vi "Add to Tree.vi"(8 "error in":errorcluster, 11 "Data in":T1) -> (0 "error out":errorcluster, 3 "Data out":T1)   [LabVIEW 2020, in "Peek Window.lvlib"]
uses:
  Peek Window.lvlib
  MHL Data Cluster.ctl
  Open Diagram Argument--cluster.ctl
  VI Types Enum.ctl
  Symbols Enum.ctl
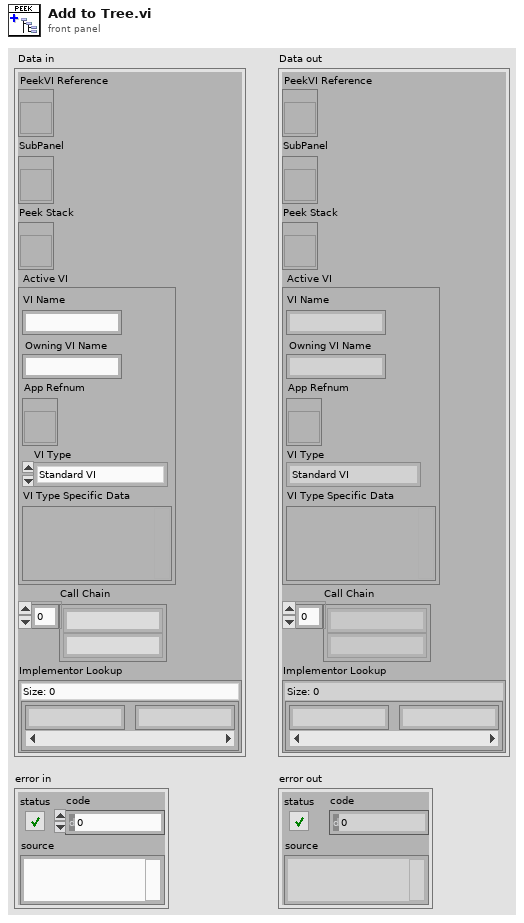
[diagram p1: front panel]
types:
  T1 = typedef "Peek Window.lvlib/MHL Data Cluster.ctl" = cluster{"PeekVI Reference":refnum<vi>, "SubPanel":refnum<vi>, "Peek Stack":refnum<vi>, "Active VI":T2, "Call Chain":string[], "Implementor Lookup":map{string, string}}
  T2 = typedef "Peek Window.lvlib/Open Diagram Argument--cluster.ctl" = cluster{"VI Name":string, "Owning VI Name":string, "App Refnum":refnum<vi>, "VI Type":T3, "VI Type Specific Data":variant}
  T3 = typedef "Peek Window.lvlib/VI Types Enum.ctl" = enum16{"Standard VI", "Dynamic Dispatch VI", "Malleable VI", "Express VI", "Polymorphic VI", "Missing VI"}
  T4 = typedef "Peek Window.lvlib/Symbols Enum.ctl" = enum16{"<Blank>", "Below Here Glyph", "VI", "Dynamic Dispatch VI", "Malleable VI", "Polymorphic VI", "Missing VI", "Express VI"}
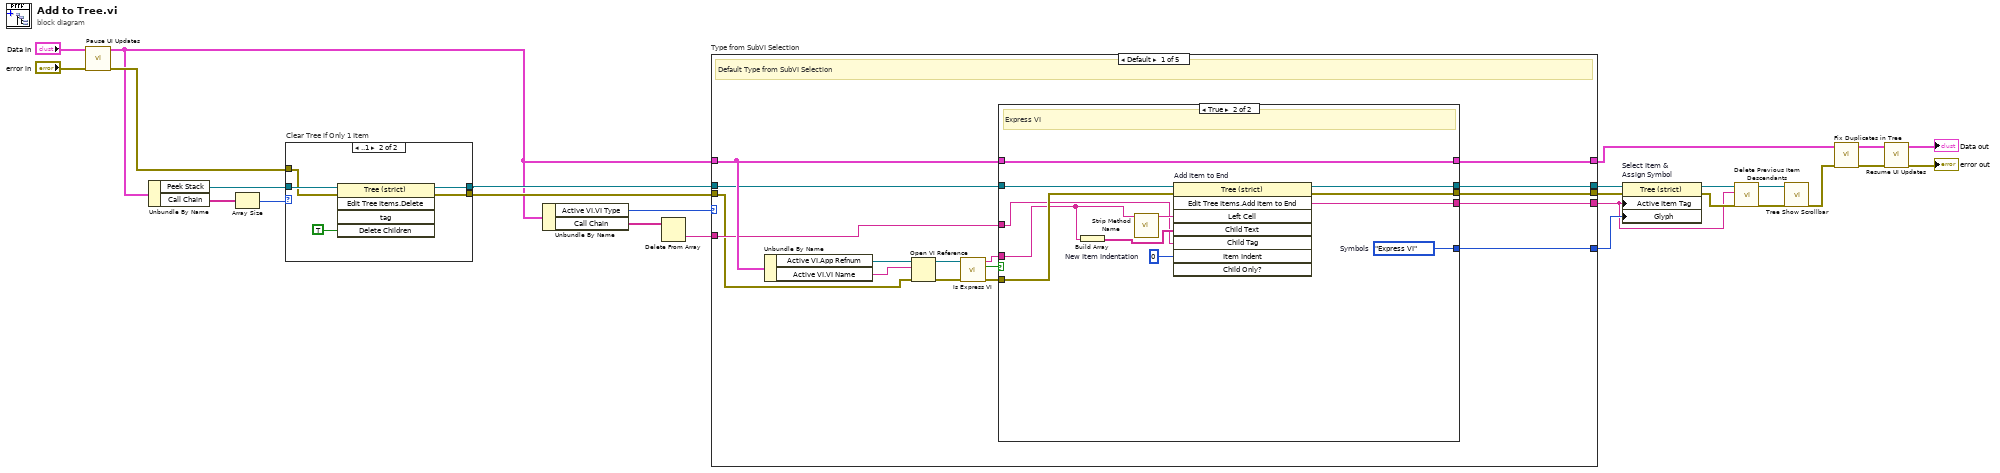
[diagram p0: block diagram]
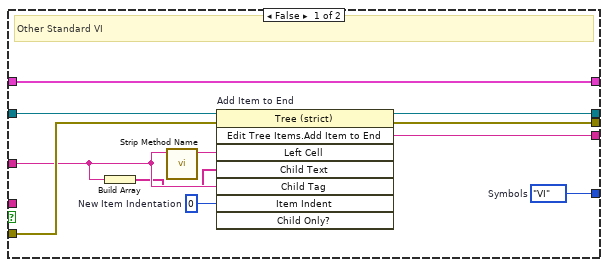
[diagram p2: hidden frame]
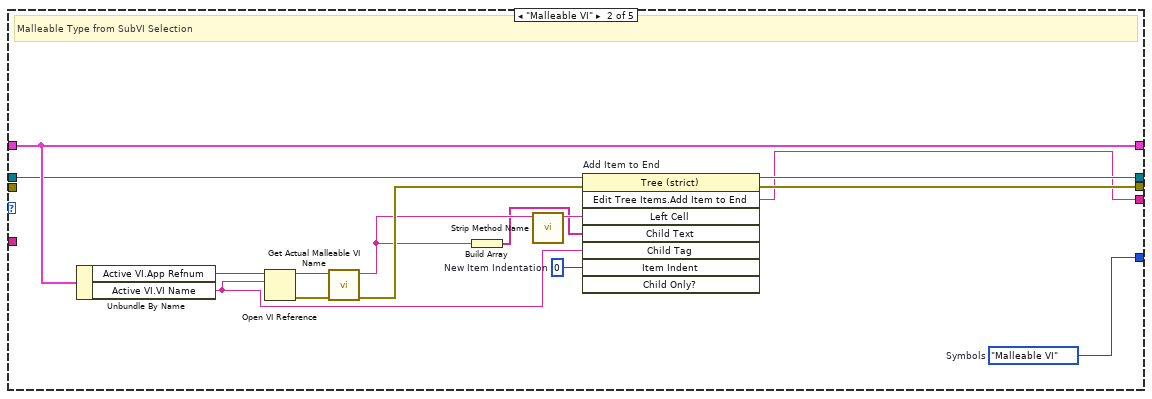
[diagram p3: hidden frame]
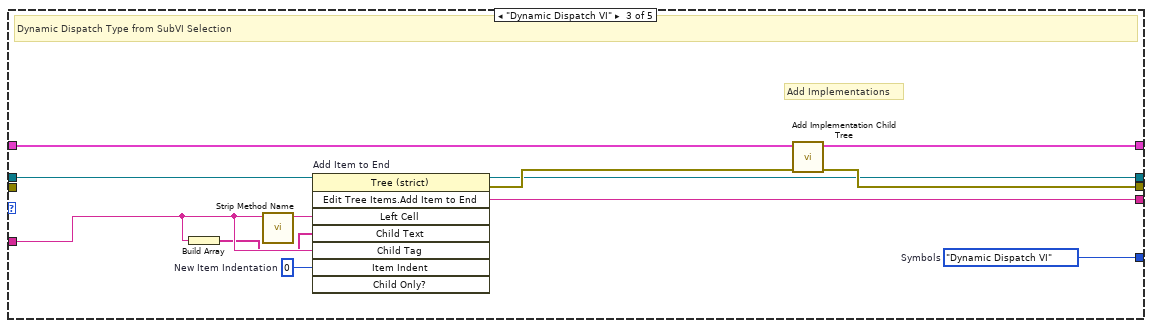
[diagram p4: hidden frame]
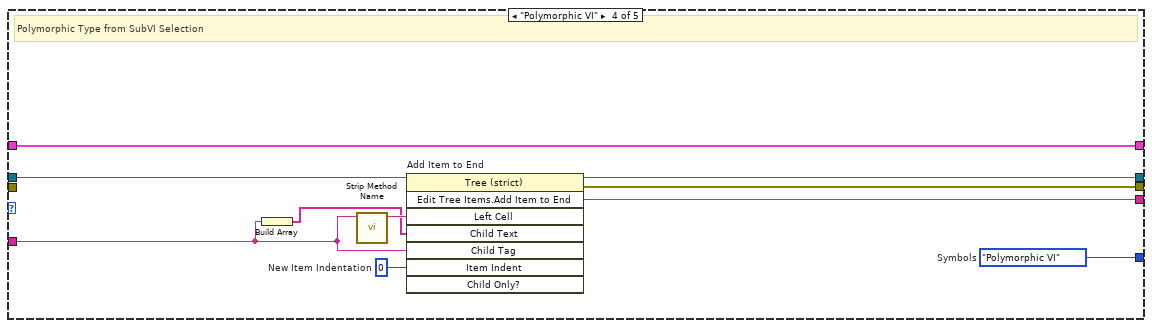
[diagram p5: hidden frame]
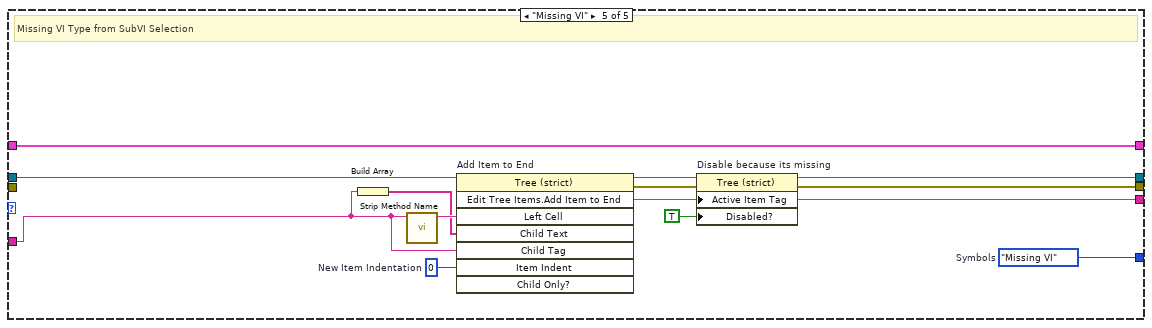
[diagram p6: hidden frame]
diagram:
  n1 = call "Pause UI Updates.vi"("error in"="error in", "Module Data"="Data in") -> ("error out"=w18:errorcluster, "Module Data"=w7:T1)  [unwired: 8 in]
  n2 = Unbundle By Name(w7) -> ("Peek Stack"=w26:refnum<vi>, "Call Chain"=w25:string[])
  n3 = Array Size(array=w25) -> (size(s)=w22:i32)
  n4 = case "Clear Tree if Only 1 Item" shown="..1" w22 {
    tunnel: w26 -> [w27 w33]
    tunnel: w18 -> [w28 w31]
    tunnel: [w28 w30] -> w8
    tunnel: [w27 w29] -> w9
    frame Default {
      # "Multiple items in call chain, add new VI to end of tree"
    }
    frame ..1 {
      # "Only one item in call chain, delete current tree and add single item"
      n5 = invoke class="Tree (strict)" method="Edit Tree Items.Delete"(reference=w33, error in=w31, "Delete Children"=TRUE ("Delete Children?")) -> (reference out=w29:refnum<vi>, error out=w30:errorcluster)  [unwired: 2 in, 3 out]
    }
  }
  n6 = Unbundle By Name(w7) -> ("Active VI.VI Type"=w5:T3, "Call Chain"=w6:string[])
  n7 = Delete From Array(array=w6) -> (deleted portion=w10:string)  [unwired: 2 in, 1 out]
  n8 = case "Type from SubVI Selection" shown="Default" w5 {
    tunnel: w7 -> [w45 w82 w96 w109 w122]
    tunnel: [w43 w77 w92 w104 w114] -> w2
    tunnel: [w44 w82 w95 w109 w122] -> w11
    tunnel: [w42 w79 w93 w105 w116] -> w3
    tunnel: w9 -> [w40 w81 w97 w106 w119]
    tunnel: w10 -> [w38 _ w89 w101 w111]
    tunnel: w8 -> [w37 _ _ _ _]
    tunnel: [w36 w80 w91 w103 w113] -> w4
    tunnel: [w35 w76 w90 w102 w112] -> w1
    frame Default {
      # "Default Type from SubVI Selection"
      n9 = Unbundle By Name(w45) -> ("Active VI.App Refnum"=w49:refnum<vi>, "Active VI.VI Name"=w39:string)
      n10 = Open VI Reference(application reference (local)=w49, vi path=w39, error in (no error)=w37) -> (vi reference=w47:refnum<vi>, error out=w48:errorcluster)  [unwired: 3 in]
      n11 = call "Is Express VI.vi"("error in"=w48, "VI Reference"=w47) -> ("error out"=w41:errorcluster, "Is Express VI"=w46:bool, "Display Name"=w34:string)  [unwired: 6 in, 1 out]
      n12 = case shown="True" w46 {
        tunnel: w45 -> [w60 w72]
        tunnel: [w60 w72] -> w44
        tunnel: [w53 w64] -> w43
        tunnel: [w56 w68] -> w42
        tunnel: w41 -> [w55 w67]
        tunnel: w40 -> [w57 w69]
        tunnel: w38 -> [w51 w61]
        tunnel: [w54 w66] -> w36
        tunnel: [w52 w65] -> w35
        tunnel: w34 -> [_ w62]
        frame False {
          w53 = Symbols_Enum."VI"  # Symbols
          w58 = 0  # New Item Indentation
          # "Other Standard VI"
          n13 = Build Array(w51) -> (w50:string[])
          n14 = call "Strip Method Name.vi"("Full Qualified Name in"=w51) -> ("Plain Method Name out"=w59:string)  [unwired: 10 in]
          n15 = invoke on="Add Item to End" class="Tree (strict)" method="Edit Tree Items.Add Item to End"(reference=w57, error in=w55, "Left Cell"=w59, "Child Text"=w50, "Child Tag"=w51, "Item Indent"=w58) -> (reference out=w54:refnum<vi>, error out=w56:errorcluster, "Edit Tree Items:Add Item to End"=w52:string)  [unwired: 2 in, 5 out]
        }
        frame True {
          w64 = Symbols_Enum."Express VI"  # Symbols
          w70 = 0  # New Item Indentation
          # "Express VI"
          n16 = Build Array(w62) -> (w63:string[])
          n17 = call "Strip Method Name.vi"("Full Qualified Name in"=w62) -> ("Plain Method Name out"=w71:string)  [unwired: 10 in]
          n18 = invoke on="Add Item to End" class="Tree (strict)" method="Edit Tree Items.Add Item to End"(reference=w69, error in=w67, "Left Cell"=w71, "Child Text"=w63, "Child Tag"=w61, "Item Indent"=w70) -> (reference out=w66:refnum<vi>, error out=w68:errorcluster, "Edit Tree Items:Add Item to End"=w65:string)  [unwired: 2 in, 5 out]
        }
      }
    }
    frame "Malleable VI" {
      w77 = Symbols_Enum."Malleable VI"  # Symbols
      w83 = 0  # New Item Indentation
      # "Malleable Type from SubVI Selection"
      n19 = Unbundle By Name(w82) -> ("Active VI.App Refnum"=w87:refnum<vi>, "Active VI.VI Name"=w75:string)
      n20 = Open VI Reference(application reference (local)=w87, vi path=w75) -> (vi reference=w86:refnum<vi>, error out=w85:errorcluster)  [unwired: 4 in]
      n21 = call "Get Actual Malleable VI Name.vi"("error in"=w85, "VI Reference"=w86) -> ("error out"=w78:errorcluster, "Malleable VI Full Qualified Name"=w74:string)  [unwired: 7 in, 1 out]
      n22 = Build Array(w74) -> (w73:string[])
      n23 = call "Strip Method Name.vi"("Full Qualified Name in"=w74) -> ("Plain Method Name out"=w84:string)  [unwired: 10 in]
      n24 = invoke on="Add Item to End" class="Tree (strict)" method="Edit Tree Items.Add Item to End"(reference=w81, error in=w78, "Left Cell"=w84, "Child Text"=w73, "Child Tag"=w75, "Item Indent"=w83) -> (reference out=w80:refnum<vi>, error out=w79:errorcluster, "Edit Tree Items:Add Item to End"=w76:string)  [unwired: 2 in, 5 out]
    }
    frame "Dynamic Dispatch VI" {
      w92 = Symbols_Enum."Dynamic Dispatch VI"  # Symbols
      w98 = 0  # New Item Indentation
      # "Add Implementations"
      # "Dynamic Dispatch Type from SubVI Selection"
      n25 = Build Array(w89) -> (w88:string[])
      n26 = call "Strip Method Name.vi"("Full Qualified Name in"=w89) -> ("Plain Method Name out"=w99:string)  [unwired: 10 in]
      n27 = invoke on="Add Item to End" class="Tree (strict)" method="Edit Tree Items.Add Item to End"(reference=w97, "Left Cell"=w99, "Child Text"=w88, "Child Tag"=w89, "Item Indent"=w98) -> (reference out=w91:refnum<vi>, error out=w94:errorcluster, "Edit Tree Items:Add Item to End"=w90:string)  [unwired: 3 in, 5 out]
      n28 = call "Add Implementation Child Tree.vi"("error in"=w94, "Data in"=w96) -> ("error out"=w93:errorcluster, "Data out"=w95:T1)  [unwired: 8 in]
    }
    frame "Polymorphic VI" {
      w104 = Symbols_Enum."Polymorphic VI"  # Symbols
      w107 = 0  # New Item Indentation
      # "Polymorphic Type from SubVI Selection"
      n29 = Build Array(w101) -> (w100:string[])
      n30 = call "Strip Method Name.vi"("Full Qualified Name in"=w101) -> ("Plain Method Name out"=w108:string)  [unwired: 10 in]
      n31 = invoke on="Add Item to End" class="Tree (strict)" method="Edit Tree Items.Add Item to End"(reference=w106, "Left Cell"=w108, "Child Text"=w100, "Child Tag"=w101, "Item Indent"=w107) -> (reference out=w103:refnum<vi>, error out=w105:errorcluster, "Edit Tree Items:Add Item to End"=w102:string)  [unwired: 3 in, 5 out]
    }
    frame "Missing VI" {
      w114 = Symbols_Enum."Missing VI"  # Symbols
      w120 = 0  # New Item Indentation
      # "Missing VI Type from SubVI Selection"
      n32 = Build Array(w111) -> (w110:string[])
      n33 = call "Strip Method Name.vi"("Full Qualified Name in"=w111) -> ("Plain Method Name out"=w121:string)  [unwired: 10 in]
      n34 = invoke on="Add Item to End" class="Tree (strict)" method="Edit Tree Items.Add Item to End"(reference=w119, "Left Cell"=w121, "Child Text"=w110, "Child Tag"=w111, "Item Indent"=w120) -> (reference out=w118:refnum<vi>, error out=w117:errorcluster, "Edit Tree Items:Add Item to End"=w112:string)  [unwired: 3 in, 5 out]
      n35 = property on="Disable because its missing" class="Tree (strict)"(reference=w118, error in=w117, "Active Item Tag"=w112, "Disabled?"=TRUE) -> (reference out=w113:refnum<vi>, error out=w116:errorcluster)
    }
  }
  n36 = property on="Select Item &\nAssign Symbol" class="Tree (strict)"(reference=w4, error in=w3, "Active Item Tag"=w1, "Glyph"=w2) -> (reference out=w24:refnum<vi>, error out=w23:errorcluster)
  n37 = call "Delete Previous Item Descendants.vi"("error in (no error)"=w23, "Edit Tree Items:Add Item to End"=w1, "TreeControl in"=w24) -> ("error out"=w12:errorcluster, "TreeControl out"=w21:refnum<vi>)  [unwired: 7 in]
  n38 = call "Tree Show Scrollbar.vi"("error in (no error)"=w12, "Tree"=w21) -> ("error out"=w14:errorcluster)  [unwired: 8 in, 1 out]
  n39 = call "Fix Duplicates in Tree.vi"("error in (no error)"=w14, "Data in"=w11) -> ("error out"=w13:errorcluster, "Data out"=w15:T1)  [unwired: 8 in]
  n40 = call "Resume UI Updates.vi"("error in"=w13, "Module Data"=w15) -> ("error out"=→"error out":errorcluster, "Module Data"=→"Data out":T1)  [unwired: 8 in]
